vi "Calculate_Gradient.vi"() -> (0 "New Values In":string[][](array[string])=[["Test data5"]], 1 "New Chs In":string[](array[string])=["30-10-03:New:Channel new5"])   [LabVIEW 2015]
uses:
  Results_plotter_Global.vi
panel:
  out "XY Graph":cluster{dbl[], dbl[]}(graph)
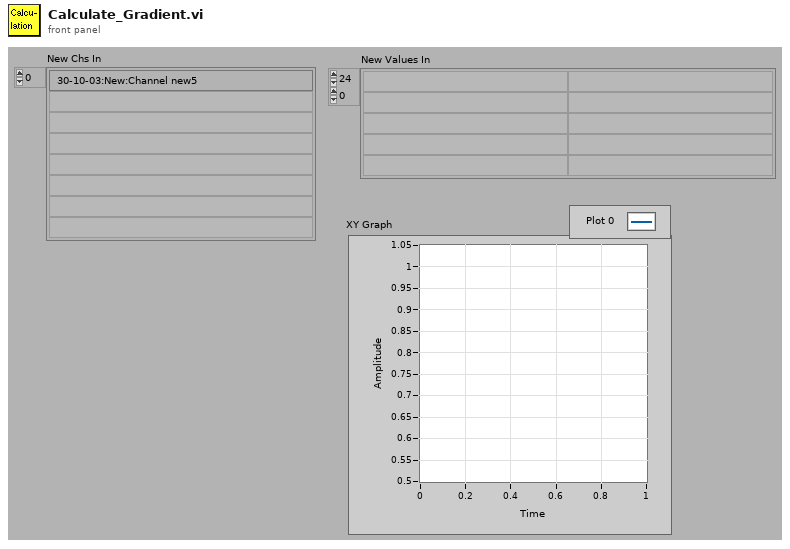
[diagram p1: front panel]
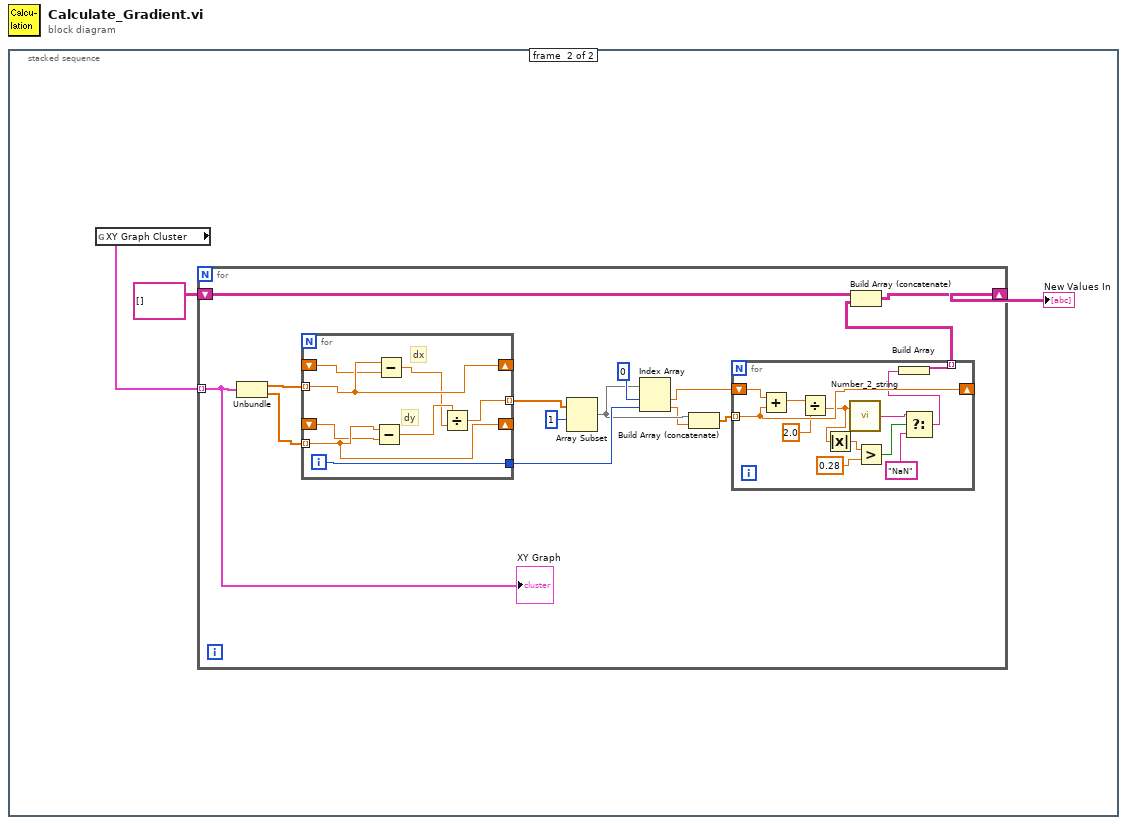
[diagram p0: block diagram]
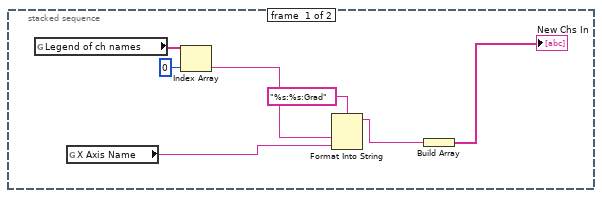
[diagram p2: hidden frame]
diagram:
  n1 = stacked-sequence {
    frame #0 {
      n2 = global read "Results_plotter_Global.vi" "Legend of ch names"() -> (w6:string[])
      n3 = global read "Results_plotter_Global.vi" "X Axis Name"() -> (w3:string)
      n4 = Index Array(array=w6, index=0) -> (element=w4:string)
      n5 = Format Into String(format string="%s:%s:Grad", w4, w3) -> (resulting string=w1:string)  [unwired: 2 in, 1 out]
      n6 = Build Array(w1) -> (→"New Chs In":string[])
    }
    frame #1 {
      n7 = global read "Results_plotter_Global.vi" "XY Graph Cluster"() -> (w10:cluster{dbl[], dbl[]}[])
      n8 = for {
        tunnel: w10 -> [w11] mode=indexing
        shift-right: [w23] -> w8
        shift-left: string[][] [] -> [w24]
        n9 = Unbundle(w11) -> (w22:dbl[], w21:dbl[])
        n10 = for {
          shift-right: [w44] -> _
          shift-left: _ -> [w43]
          shift-right: [w42] -> _
          shift-left: _ -> [w41]
          tunnel: w22 -> [w44] mode=indexing
          tunnel: w21 -> [w42] mode=indexing
          tunnel: [w38] -> w19 mode=indexing
          tunnel: [w37] -> w17
          i -> [w37]
          # "dy"
          # "dx"
          n11 = Subtract(x=w42, y=w41) -> (x-y=w40:dbl)
          n12 = Subtract(x=w44, y=w43) -> (x-y=w39:dbl)
          n13 = Divide(x=w40, y=w39) -> (x/y=w38:dbl)
        }
        n14 = Array Subset(array=w19, index=1) -> (w15:dbl[])  [unwired: 1 in]
        n15 = Index Array(array=w15, index #1=0 ("index"), index #2=w17) -> (element #1=w18:dbl, element #2=w14:dbl)
        n16 = Build Array (concatenate)(w15, w14) -> (w13:dbl[])
        n17 = for {
          shift-right: [w35] -> _
          shift-left: w18 -> [w36]
          tunnel: w13 -> [w35] mode=indexing
          tunnel: [w32] -> w12 mode=indexing
          n18 = Add(x=w36, y=w35) -> (x+y=w34:dbl)
          n19 = Divide(x=w34, y=2.0) -> (x/y=w26:dbl)
          n20 = Absolute Value(x=w26) -> (abs(x)=w25:dbl)
          n21 = call "Number_2_string.vi"("number"=w26) -> ("String"=w29:string)  [unwired: 1 in]
          n22 = Greater?(x=w25, y=0.28) -> (0:w30:bool)
          n23 = Select(t=w29, s=w30, f="NaN") -> (s? t:f=w28:string)
          n24 = Build Array(w28) -> (w32:string[])
        }
        n25 = Build Array (concatenate)(w24, w12) -> (w23:string[][])
        "XY Graph" <- w11
      }
      "New Values In" <- w8
    }
  }
